vi "Error VI.vi"(8 "error in (no error)":errorcluster) -> ()   [LabVIEW 2009, in "PXI-4130 Custom Device.lvlib"]
uses:
  PXI-4130 Custom Device.lvlib
  <vilib>/NI_Real-Time Target Support.lvlib
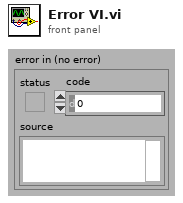
[diagram p1: front panel]
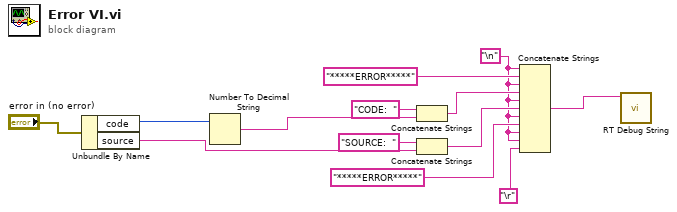
[diagram p0: block diagram]
diagram:
  w2 = "\n"
  n1 = Unbundle By Name("error in (no error)") -> ("code"=w12:i32, "source"=w6:string)
  n2 = Number To Decimal String(number=w12) -> (decimal integer string=w9:string)  [unwired: 1 in]
  n3 = Concatenate Strings("CODE:  " ("string"), w9) -> (w8:string)
  n4 = Concatenate Strings("SOURCE:  " ("string"), w6) -> (w5:string)
  n5 = Concatenate Strings(w2, "*****ERROR*****" ("string"), w2, w8, w2, w5, w2, "*****ERROR*****" ("string"), w2, w2, "\r") -> (w4:string)
  n6 = call <vilib>:"RT Debug String.vi"("String to write"=w4) -> ()  [unwired: 10 in, 1 out]
